vi "Scan_test1.vi"   [LabVIEW 2020]
uses:
  <vilib>/Platform/TimedLoop/XDataNode/timing_clust.ctl
  <vilib>/Platform/TimedLoop/XDataNode/nitl_modes.ctl
  <vilib>/Platform/TimedLoop/XDataNode/wakeup.ctl
  <vilib>/rvi/Emulation/niFpgaSctlEmulationGetInTimedLoop.vi
  <vilib>/rvi/Emulation/niFpgaEmulationReportErrorSimple.vi
  <vilib>/rvi/Emulation/niFpgaGetClockAttributes.vi
  <vilib>/rvi/Emulation/niFpgaCriticalErrorInLSC.vi
  <vilib>/rvi/eio/common/nirviEmuTemplateMethod_errors.vi
  <vilib>/Platform/TimedLoop/XDataNode/XDataNode.xnode
  <vilib>/eio/EIONode/EIONode.xnode
  <vilib>/Platform/TimedLoop/XDataNode/XDNodeRunTimeDep.lvlib
types:
  T1 = typedef "XDNodeRunTimeDep.lvlib/timing_clust.ctl" = cluster{"Expected End [f-1]":u64, "Actual End [f-1]":u64, "Finished Late? [f-1]":bool, "Expected End [i-1]":u64, "Actual End [i-1]":u64, "Finished Late? [i-1]":bool, "Expected Start [i]":u64, "Actual Start [i]":u64, "Expected Start [f]":u64, "Actual Start [f]":u64, "Source Name":string, "Structure Name":string, "Period":i64, "Deadline":i64, "Offset":i64, "Start":i64, "Priority":i32, "Timeout":i32, "Mode":T2, "Wakeup Reason":T3, "Error":errorcluster, "Source Type":string, "Secondary Source Type":string, "Global End Time":u64, "Global Start Time":u64, "Frame Duration":u64, "Iteration Duration":u64, "Assigned CPU":i32, "I/O Scan Engine Mode":u32}
  T2 = typedef "XDNodeRunTimeDep.lvlib/nitl_modes.ctl" = enum32{"No Change", "Process missed periods, maintain original phase", "Discard missed periods, maintain original phase", "Process missed periods, ignore original phase", "Discard missed periods, ignore original phase"}
  T3 = typedef "XDNodeRunTimeDep.lvlib/wakeup.ctl" = enum32{"Normal", "Aborted", "Asynchronous wakeup", "Timing source error", "Timed loop error", "Timeout"}
  T4 = cluster{"Enable":bool, "Polarity":bool, "Period":u32, "PulseWidth":u32}
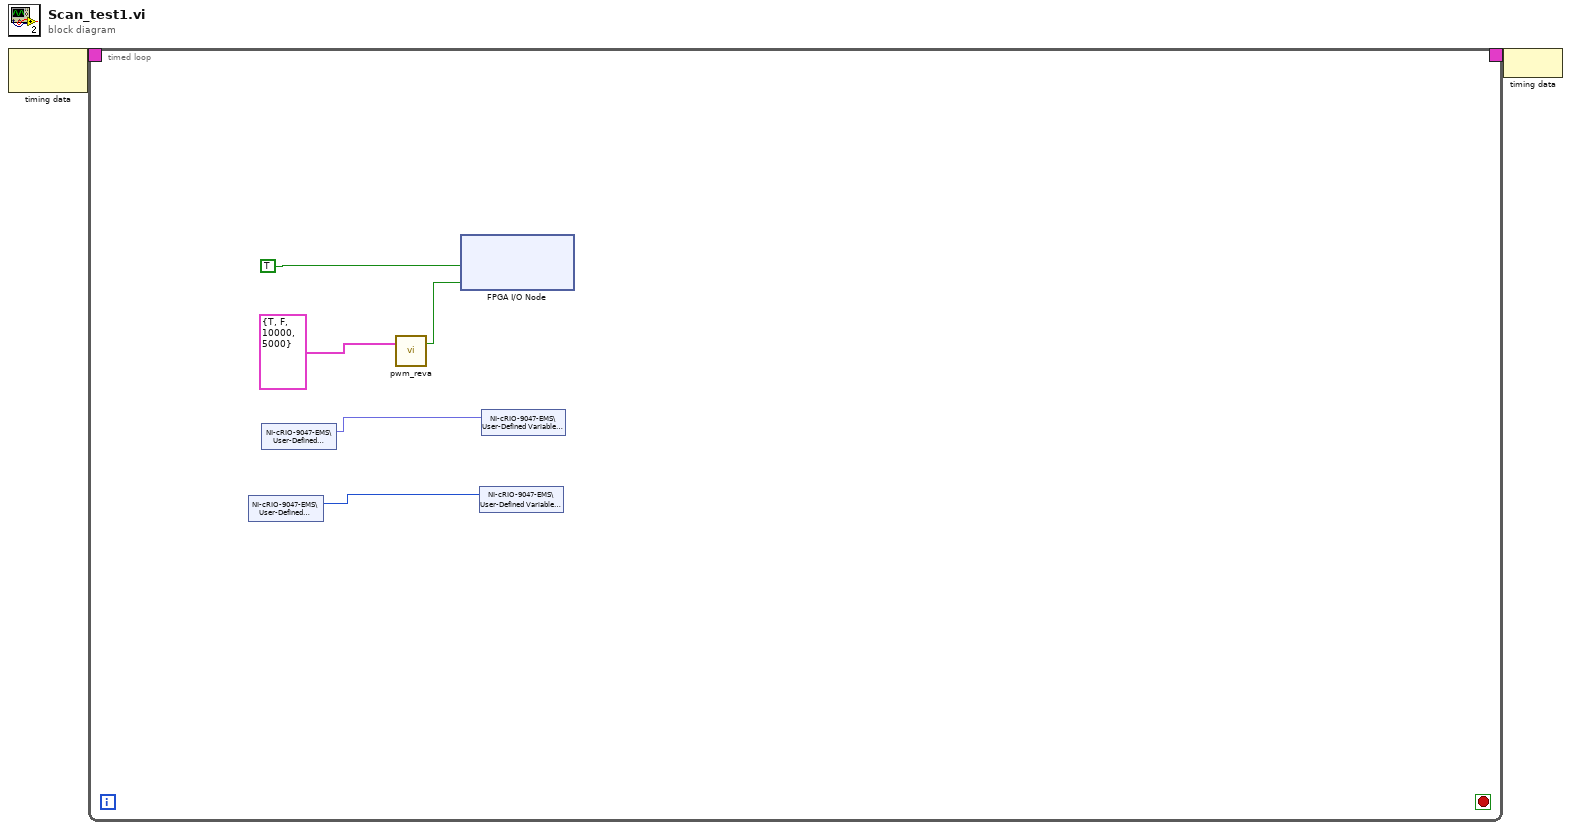
[diagram p0: block diagram]
diagram:
  n1 = node-c288() -> (w2:T1)  [unwired: 1 in]
  n2 = timed-loop {
    timing: w2 -> [_]
    timing-out: [_] -> w1
    stop <- _ stop-if-true
    n3 = shared-variable "NI-cRIO-9047-EMS\\User-Defined Variables\\Int_in"() -> (w5:i32)  [unwired: 1 in, 1 out]
    n4 = shared-variable "NI-cRIO-9047-EMS\\User-Defined Variables\\Fix_in"() -> (w6:fxp<+/-,32,16>)  [unwired: 1 in, 1 out]
    n5 = call <vilib>:"pwm_reva.vi"("PWMControl"=T4 {"Enable"=TRUE, "Polarity"=FALSE, "Period"=10000, "PulseWidth"=5000}) -> ("OutSig"=w3:bool)  [unwired: 2 in]
    n6 = xnode "FPGA I/O Node"("Mod6/DIO0"=TRUE, "Mod6/DIO1"=w3) -> ()  [unwired: 2 in, 2 out]
    n7 = shared-variable "NI-cRIO-9047-EMS\\User-Defined Variables\\Int_out"(w5) -> ()  [unwired: 1 in, 1 out]
    n8 = shared-variable "NI-cRIO-9047-EMS\\User-Defined Variables\\Fix_out"(w6) -> ()  [unwired: 1 in, 1 out]
  }
  n9 = node-c288(w1) -> ()
